vi "Sort tree items.vi"(11 "Array":string[][](array[string])) -> (3 "sorted 2D array":string[][](array[string]))   [LabVIEW 2025, in "CAN-LIN Raw Bus Capture UI.lvlib"]
uses:
  CAN-LIN Raw Bus Capture UI.lvlib
  93072385-aadc-4cbd-bce5-5c3ccd734ba2.vi
  <vilib>/Array/Sort 2D Array - Pop Stack.vi
  <vilib>/Array/Sort 2D Array - Push Stack.vi
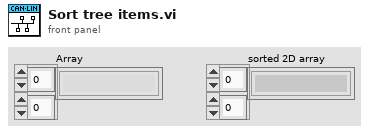
[diagram p1: front panel]
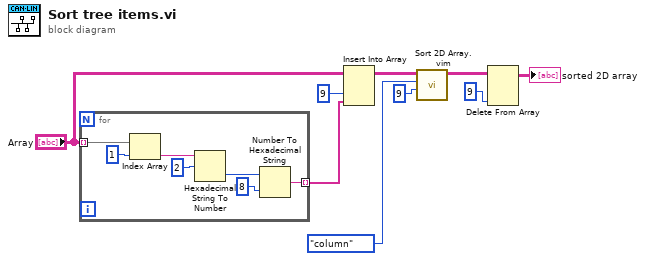
[diagram p0: block diagram]
diagram:
  n1 = for {
    tunnel: [w12] -> w3 mode=indexing
    tunnel: "Array" -> [w10] mode=indexing
    n2 = Index Array(array=w10, index=1 ("index (row)")) -> (element=w15:string)
    n3 = Hexadecimal String To Number(string=w15, offset=2) -> (number=w13:u32)  [unwired: 1 in, 1 out]
    n4 = Number To Hexadecimal String(1:i16 8 ("width (-)"), 2:w13) -> (0:w12:string)
  }
  n5 = Insert Into Array(array="Array", index (col)=9, new element=w3) -> (w4:string[][])  [unwired: 1 in]
  n6 = call "Sort 2D Array.vim"("index"=9, "dimension to index (column)"=enum16{"column", "row"}."column", "2D array"=w4) -> ("sorted 2D array"=w7:string[][])  [unwired: 7 in, 1 out]
  n7 = Delete From Array(array=w7, index (col)=9) -> (array with subset deleted=→"sorted 2D array":string[][])  [unwired: 2 in, 1 out]
